vi "Generate grid.vi"(0 "Spots x":i32, 1 "Spots y":i32, 2 "Grid spacing":i32) -> (3 "X":i32[](array[numeric]), 4 "Y":i32[](array[numeric]), 5 "Z":i32[](array[numeric]), 6 "I":i32[](array[numeric]))   [LabVIEW 2011]
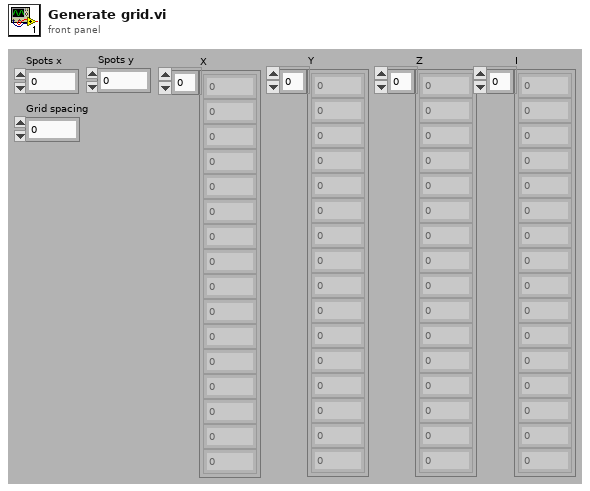
[diagram p1: front panel]
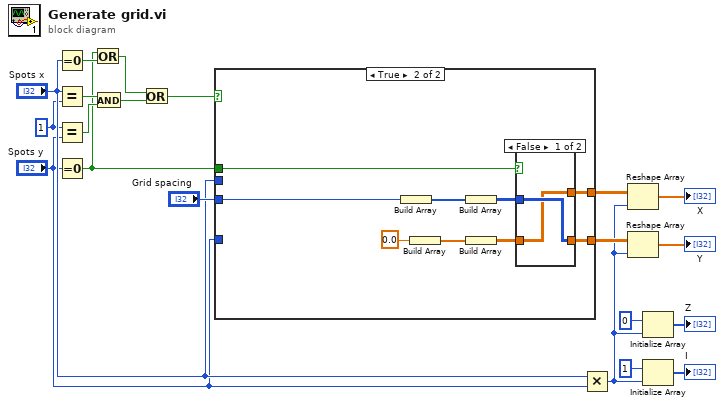
[diagram p0: block diagram]
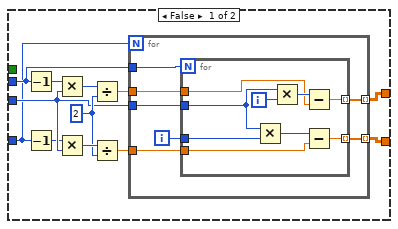
[diagram p2: hidden frame]
diagram:
  w5 = 1 ("y")
  n1 = Equal To 0?(x="Spots x") -> (x = 0?=w10:bool)
  n2 = Equal?(x="Spots x", y=w5) -> (x = y?=w3:bool)
  n3 = Equal?(x=w5, y="Spots y") -> (x = y?=w2:bool)
  n4 = Equal To 0?(x="Spots y") -> (x = 0?=w1:bool)
  n5 = Or(x=w1, y=w10) -> (x .or. y?=w9:bool)
  n6 = And(x=w3, y=w2) -> (x .and. y?=w7:bool)
  n7 = Or(x=w9, y=w7) -> (x .or. y?=w8:bool)
  n8 = case shown="True" w8 {
    tunnel: [w27 w49] -> w20
    tunnel: "Grid spacing" -> [w26 w56]
    tunnel: [w23 w53] -> w16
    tunnel: "Spots x" -> [w22 _]
    tunnel: w1 -> [_ w57]
    tunnel: "Spots y" -> [w21 _]
    frame False {
      w30 = 2 ("y")
      n9 = Decrement(x=w22) -> (x-1=w24:i32)
      n10 = Decrement(x=w21) -> (x-1=w25:i32)
      n11 = Multiply(x=w24, y=w26) -> (x*y=w31:i32)
      n12 = Multiply(x=w25, y=w26) -> (x*y=w32:i32)
      n13 = Divide(x=w31, y=w30) -> (x/y=w29:dbl)
      n14 = Divide(x=w32, y=w30) -> (x/y=w28:dbl)
      n15 = for {
        N: w21 -> [_]
        tunnel: w22 -> [w39]
        tunnel: w26 -> [w37]
        tunnel: w29 -> [w36]
        tunnel: w28 -> [w35]
        tunnel: [w34] -> w27 mode=indexing
        tunnel: [w33] -> w23 mode=indexing
        i -> [w38]
        n16 = for {
          N: w39 -> [_]
          tunnel: w38 -> [w47]
          tunnel: w37 -> [w46]
          tunnel: w36 -> [w44]
          tunnel: w35 -> [w42]
          tunnel: [w41] -> w34 mode=indexing
          tunnel: [w40] -> w33 mode=indexing
          i -> [w48]
          n17 = Multiply(x=w46, y=w47) -> (x*y=w43:i32)
          n18 = Multiply(x=w46, y=w48) -> (x*y=w45:i32)
          n19 = Subtract(x=w45, y=w44) -> (x-y=w41:dbl)
          n20 = Subtract(x=w43, y=w42) -> (x-y=w40:dbl)
        }
      }
    }
    frame True {
      n21 = Build Array(w56) -> (w55:i32[])
      n22 = Build Array(0.0 ("element")) -> (w52:dbl[])
      n23 = Build Array(w55) -> (w54:i32[][])
      n24 = Build Array(w52) -> (w50:dbl[][])
      n25 = case shown="False" w57 {
        tunnel: w54 -> [w59 w61]
        tunnel: [w59 w60] -> w53
        tunnel: w50 -> [w58 w60]
        tunnel: [w58 w61] -> w49
        frame False {
        }
        frame True {
        }
      }
    }
  }
  n26 = Multiply(x="Spots x", y="Spots y") -> (x*y=w12:i32)
  n27 = Reshape Array(w20, w12) -> (→"X":dbl[])
  n28 = Reshape Array(w16, w12) -> (→"Y":dbl[])
  n29 = Initialize Array(0 ("element"), w12) -> (→"Z":i32[])
  n30 = Initialize Array(1 ("element"), w12) -> (→"I":i32[])
